vi "Write Range.vi"(8 "error in (no error)":errorcluster, 10 "Range":dbl, 11 "DMM in":refnum<class "DMM.lvclass">) -> (0 "error out":errorcluster, 3 "DMM out":refnum<class "DMM.lvclass">)   [LabVIEW 2020, in "DMM.lvclass"]
uses:
  DMM.lvclass
  DMM.lvclass/DMM.ctl
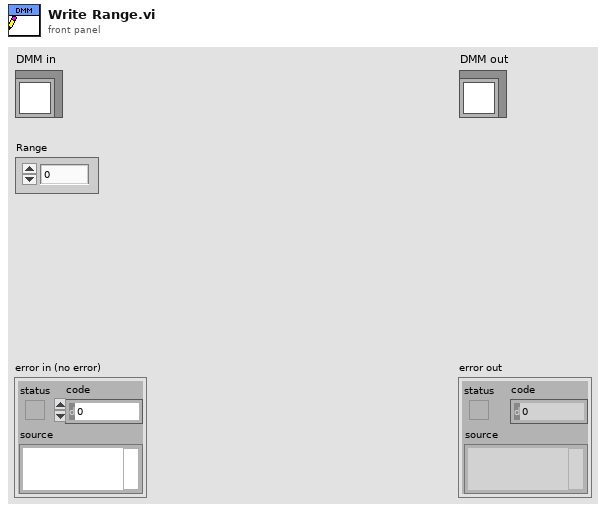
[diagram p1: front panel]
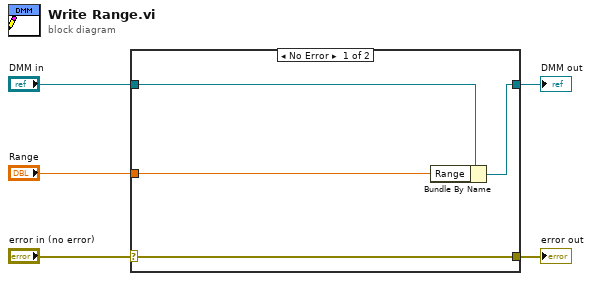
[diagram p0: block diagram]
diagram:
  n1 = case shown="No Error" "error in (no error)" {
    selector: "error in (no error)" -> [w9 w10]
    tunnel: [w9 w10] -> w4
    tunnel: [w7 w11] -> w2
    tunnel: "DMM in" -> [w8 w11]
    tunnel: "Range" -> [w6 _]
    frame No Error {
      n2 = Bundle By Name(cluster=w8, "Range"=w6) -> (w7:refnum<class "DMM.lvclass">)
    }
    frame Error {
    }
  }
  "error out" <- w4
  "DMM out" <- w2
